vi "例4-15.vi"() -> ()   [LabVIEW 2019]
panel:
  out "学生簇":T1
  in  "年龄":dbl=18.0
  in  "性别":string="男"
  in  "姓名":string="李大山"
  in  "学号":u32=201904012
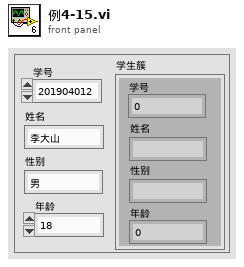
[diagram p1: front panel]
types:
  T1 = cluster{"学号":u32, "姓名":string, "性别":string, "年龄":dbl}
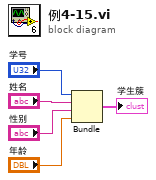
[diagram p0: block diagram]
diagram:
  n1 = Bundle("学号"="学号", "姓名"="姓名", "性别"="性别", "年龄"="年龄") -> (→"学生簇":T1)  [unwired: 1 in]
